vi "Configure DAQ Trigger (Marker0 to PFI).vi"(8 "error in (no error)":errorcluster, 9 "FGEN Channels":string[](array[string]), 10 "FGEN Resource":refnum<k15>, 11 "DAQmx Tasks In":T2) -> (0 "error out":errorcluster, 2 "FGEN-DAQ Routing":T1, 3 "DAQmx Tasks Out":T2)   [LabVIEW 2025]
uses:
  <vilib>/DAQmx/configure/trigger.llb/DAQmx Start Trigger (Digital Edge).vi
  <resource>/objmgr/daqmx.rc
  <instrlib>/niFgen/niFgen.llb/niFgen_ctl Exported Signal Identifiers (Ring).ctl
  <instrlib>/niFgen/niFgen.llb/niFgen_ctl Exported Signal Name Values (Ring).ctl
  <instrlib>/niFgen/niFgen.llb/niFgen_ctl Exported Signal Desination Values (ComboBox).ctl
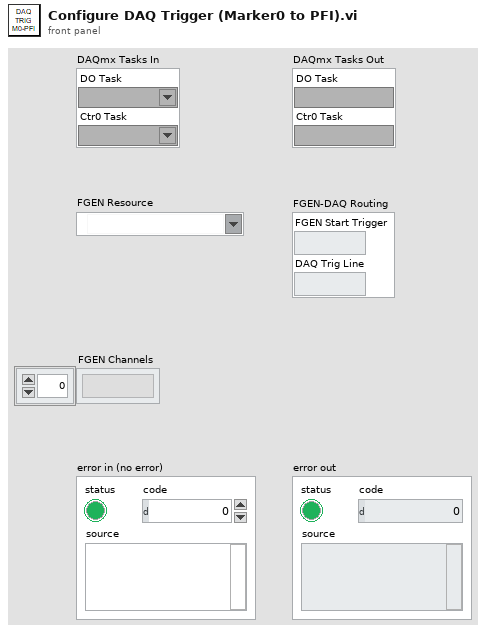
[diagram p1: front panel]
types:
  T1 = cluster{"FGEN Start Trigger":string, "DAQ Trig Line":string}
  T2 = cluster{"DO Task":refnum<k21>, "Ctr0 Task":refnum<k21>}
  T3 = typedef "niFgen_ctl Exported Signal Desination Values (ComboBox).ctl" = string
  T4 = typedef "niFgen_ctl Exported Signal Identifiers (Ring).ctl" = string
  T5 = typedef "niFgen_ctl Exported Signal Name Values (Ring).ctl" = u16
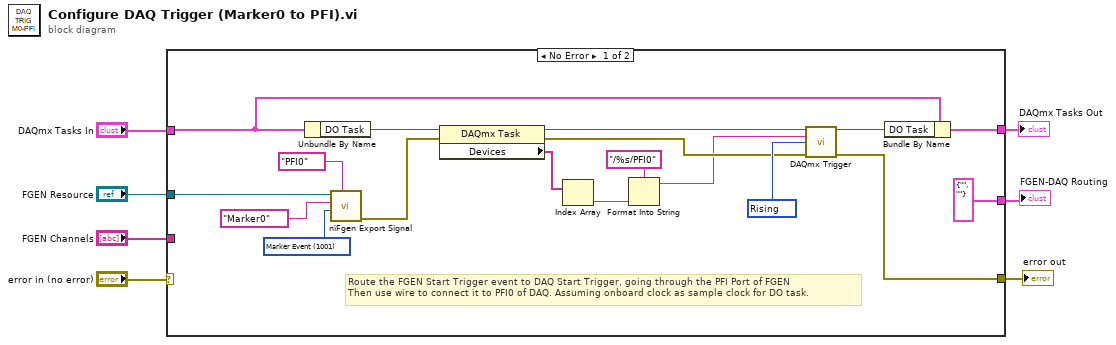
[diagram p0: block diagram]
diagram:
  n1 = case shown="No Error" "error in (no error)" {
    selector: "error in (no error)" -> [_ w26]
    tunnel: [w22 w26] -> w7
    tunnel: "DAQmx Tasks In" -> [w20 _]
    tunnel: [w21 _] -> w4
    tunnel: "FGEN Resource" -> [w13 _]
    tunnel: "FGEN Channels" -> [_ _]
    tunnel: [T1 {"FGEN Start Trigger"="", "DAQ Trig Line"=""} ("FGEN-DAQ Routing") _] -> w1
    frame No Error {
      w11 = T5 1001 items=["Sample Clock"=101, "Sample Clock Timebase"=1006, "Reference Clock"=102, "Onboard Reference Clock"=1019, "Start Trigger"=1004, "Script Trigger"=103, "Marker Event"=1001, "Data Marker Event"=108, "Ready For Start Event"=105, "Started Event"=106, "Done Event"=107, "Synchronization Pulse"=1007, "Sync Out"=1002] ("Signal")
      w24 = 10280 items=["Rising"=10280, "Falling"=10171] ("edge")
      # "Route the FGEN Start Trigger event to DAQ Start Trigger, going through the PFI Port of FGEN\nThen use wire to connect it to PFI0 of DAQ. Assuming onboard clock as sample clock for DO task."
      n2 = Unbundle By Name(w20) -> ("DO Task"=w23:refnum<k21>)
      n3 = call <instrlib>:"niFgen Export Signal.vi"("Output Terminal (do not export)"=T3 "PFI0", "Signal"=w11, "Signal Identifier (None)"=T4 "Marker0", "Instrument Handle"=w13) -> ("error out"=w8:errorcluster)  [unwired: 6 in, 1 out]
      n4 = property class="DAQmx Task"(reference=w23, error in=w8) -> (reference out=w19:refnum<k21>, error out=w15:errorcluster, "Devices"=w18:tag[])
      n5 = Index Array(array=w18) -> (element=w16:tag)  [unwired: 1 in]
      n6 = Format Into String(format string="/%s/PFI0", w16) -> (resulting string=w14:string)  [unwired: 2 in, 1 out]
      n7 = call-poly <vilib>:"DAQmx Trigger.vi"("task/channels in"=w19, "source"=w14, "edge"=w24, "error in"=w15) -> ("task out"=w25:refnum<k21>, "error out"=w22:errorcluster)  [unwired: 10 in]
      n8 = Bundle By Name(cluster=w20, "DO Task"=w25) -> (w21:T2)
    }
    frame Error {
    }
  }
  "error out" <- w7
  "DAQmx Tasks Out" <- w4
  "FGEN-DAQ Routing" <- w1
